vi "Do 6-Contact Sample Resistivity Calculations.vi"(8 "error in (no error)":errorcluster) -> (0 "error out":errorcluster)   [LabVIEW 2016, in "Hall Effect Library.lvlib"]
uses:
  Hall Effect Library.lvlib
  Global Variables/Hall Effect Data.vi
  Global Variables/Test Settings.vi
panel:
  out "PAvg":dbl
  out "PB":dbl
  out "PA":dbl
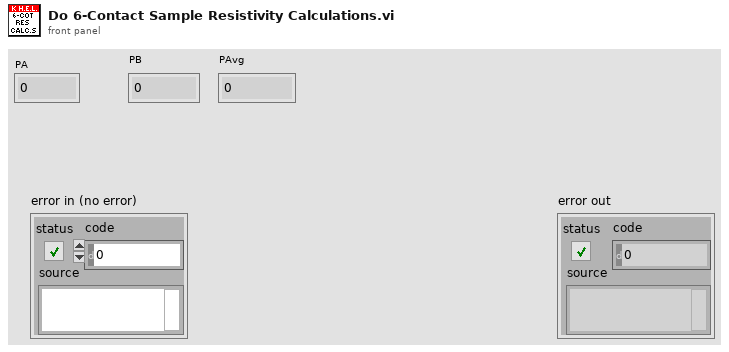
[diagram p1: front panel]
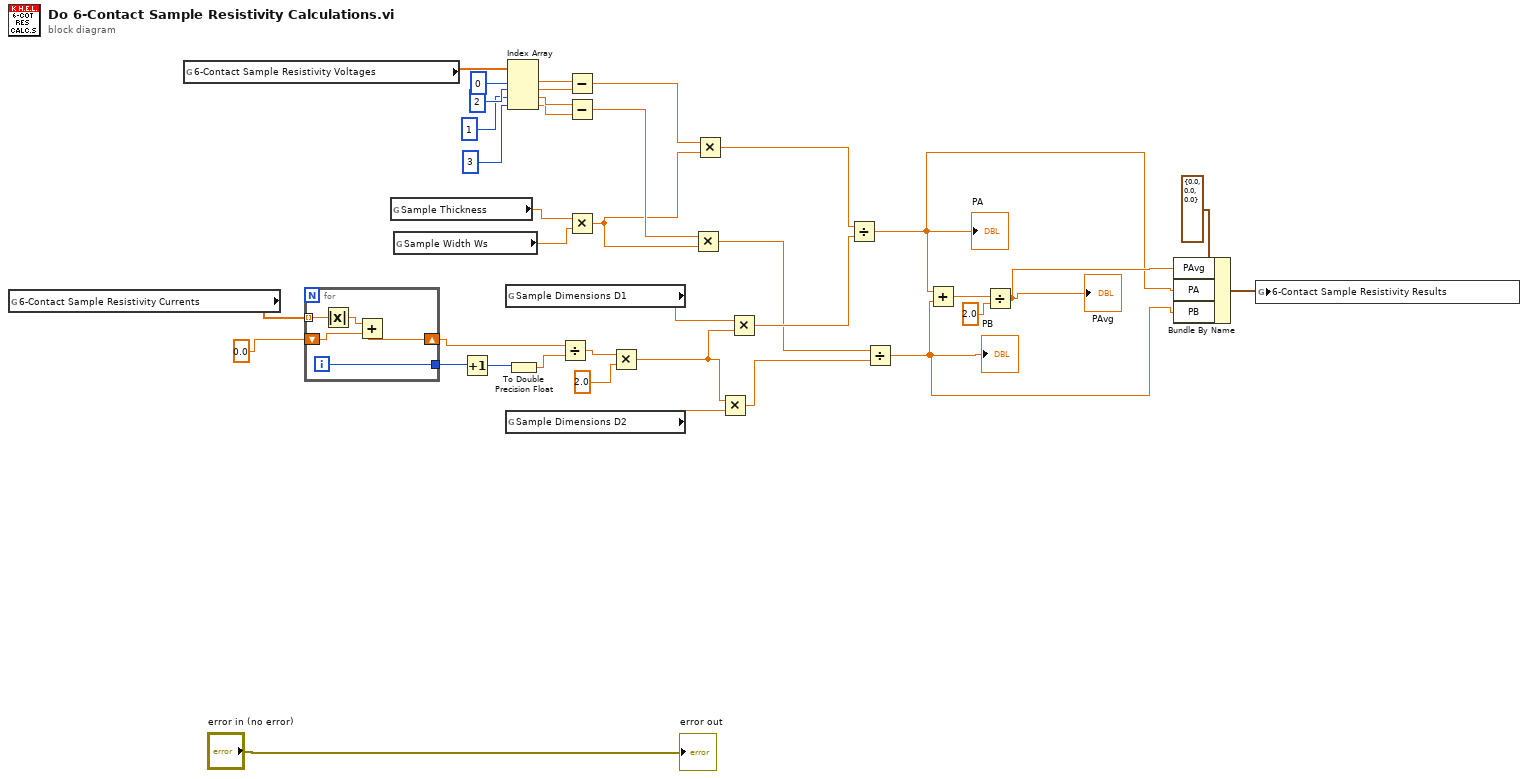
[diagram p0: block diagram]
diagram:
  n1 = global read "Hall Effect Data.vi" "6-Contact Sample Resistivity Currents"() -> (w35:dbl[])
  n2 = global read "Hall Effect Data.vi" "6-Contact Sample Resistivity Voltages"() -> (w30:dbl[])
  n3 = for {
    shift-right: [w41] -> w32
    shift-left: 0.0 -> [w42]
    tunnel: w35 -> [w39] mode=indexing
    tunnel: [w40] -> w34
    i -> [w40]
    n4 = Absolute Value(x=w39) -> (abs(x)=w38:dbl)
    n5 = Add(x=w38, y=w42) -> (x+y=w41:dbl)
  }
  n6 = global read "Test Settings.vi" "Sample Thickness"() -> (w21:dbl)
  n7 = global read "Test Settings.vi" "Sample Width Ws"() -> (w20:dbl)
  n8 = Increment(x=w34) -> (x+1=w33:i32)
  n9 = global read "Test Settings.vi" "Sample Dimensions D1"() -> (w14:dbl)
  n10 = global read "Test Settings.vi" "Sample Dimensions D2"() -> (w12:dbl)
  n11 = Index Array(array=w30, index #1=0, index #2=2, index #3=1, index #4=3) -> (element #1=w25:dbl, element #2=w24:dbl, element #3=w23:dbl, element #4=w22:dbl)
  n12 = To Double Precision Float(number=w33) -> (double precision float=w31:dbl)
  n13 = Divide(x=w32, y=w31) -> (x/y=w16:dbl)
  n14 = Subtract(x=w25, y=w24) -> (x-y=w19:dbl)
  n15 = Subtract(x=w23, y=w22) -> (x-y=w18:dbl)
  n16 = Multiply(x=w21, y=w20) -> (x*y=w17:dbl)
  n17 = Multiply(x=w16, y=2.0) -> (x*y=w13:dbl)
  n18 = Multiply(x=w18, y=w17) -> (x*y=w9:dbl)
  n19 = Multiply(x=w19, y=w17) -> (x*y=w11:dbl)
  n20 = Multiply(x=w13, y=w12) -> (x*y=w8:dbl)
  n21 = Multiply(x=w14, y=w13) -> (x*y=w10:dbl)
  n22 = Divide(x=w11, y=w10) -> (x/y=w3:dbl)
  "PA" <- w3
  n23 = Divide(x=w9, y=w8) -> (x/y=w2:dbl)
  "PB" <- w2
  n24 = Add(x=w3, y=w2) -> (x+y=w7:dbl)
  n25 = Divide(x=w7, y=2.0) -> (x/y=w4:dbl)
  "PAvg" <- w4
  n26 = Bundle By Name(cluster=cluster{"PAvg":dbl, "PA":dbl, "PB":dbl} {"PAvg"=0.0, "PA"=0.0, "PB"=0.0} ("6-Contact Sample Resistivity Results"), "PAvg"=w4, "PA"=w3, "PB"=w2) -> (w1:cluster{"PAvg":dbl, "PA":dbl, "PB":dbl})
  n27 = global write "Hall Effect Data.vi" "6-Contact Sample Resistivity Results"(w1) -> ()
  "error out" <- "error in (no error)"
